vi "Init.vi"(0 "error in (no error)":errorcluster) -> (1 "IGxFactory":refnum<k24>, 2 "error out":errorcluster)   [LabVIEW 2013, in "GxLVlib.lvlib"]
uses:
  GxLVlib.lvlib
  F:/GxILibrary/Labview/trunk/private/dev/src/C#/x86/GxLVLib/dll/GxIAPINET.dll
  private/dev/src/C#/x86/GxLVLib/dll/GxIAPINET.dll
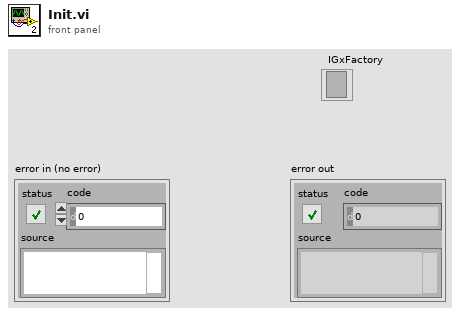
[diagram p1: front panel]
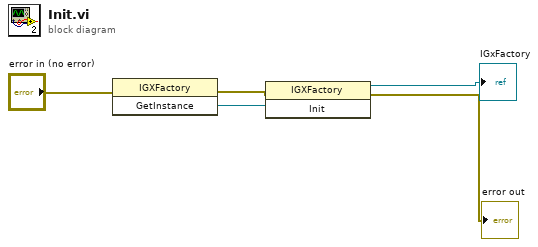
[diagram p0: block diagram]
diagram:
  n1 = invoke class="IGXFactory" method="GetInstance"(error in="error in (no error)") -> (error out=w3:errorcluster, "GetInstance"=w4:refnum<k24>)  [unwired: 2 in, 1 out]
  n2 = invoke class="IGXFactory" method="Init"(reference=w4, error in=w3) -> (reference out=→"IGxFactory":refnum<k24>, error out=→"error out":errorcluster)  [unwired: 1 in, 1 out]
